vi "Test Data 2.vi"(8 "error in (no error)":errorcluster, 11 "Instrument.Lockin in":refnum<class "Instrument.Lockin.lvclass">) -> (0 "error out":errorcluster, 3 "Instrument.Lockin out":refnum<class "Instrument.Lockin.lvclass">)   [LabVIEW 2019]
uses:
  src/Instrument.Lockin/Instrument.Lockin.lvclass
  <vilib>/addons/_JKI Toolkits/Caraya/classes/Test/Test.lvclass
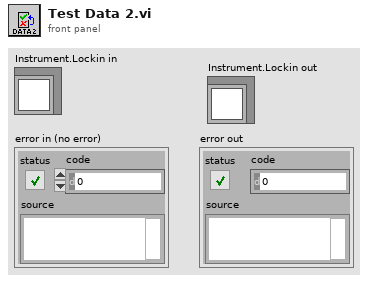
[diagram p1: front panel]
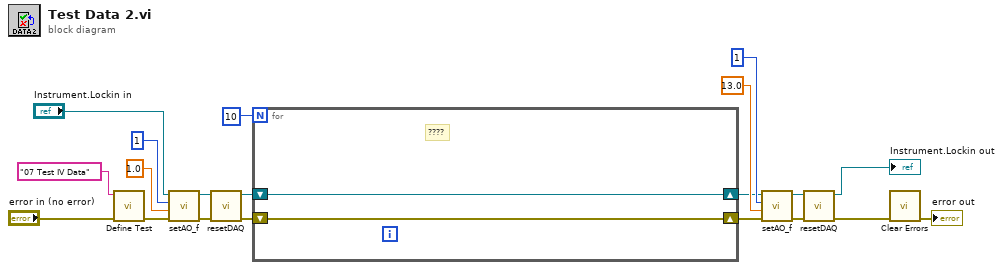
[diagram p0: block diagram]
diagram:
  n1 = call <vilib>:"Define Test.vi"("error in (no error)"="error in (no error)", "Label (VI Title)"="07 Test IV Data") -> ("error out"=w17:errorcluster)  [unwired: 8 in, 1 out]
  n2 = call-dynamic "setAO_f.vi"("error in (no error)"=w17, "Frequency (Hz)"=1.0, "AO Channel"=1, "Instrument.Lockin in"="Instrument.Lockin in") -> ("error out"=w9:errorcluster, "Instrument.Lockin out"=w8:refnum<class "Instrument.Lockin.lvclass">)  [unwired: 6 in]
  n3 = call-dynamic "resetDAQ.vi"("error in (no error)"=w9, "Instrument.Lockin in"=w8) -> ("error out"=w7:errorcluster, "Instrument.Lockin out"=w6:refnum<class "Instrument.Lockin.lvclass">)  [unwired: 8 in]
  n4 = for {
    N: 10 -> [_]
    shift-right: [w21] -> w11
    shift-left: w7 -> [w21]
    shift-right: [w22] -> w10
    shift-left: w6 -> [w22]
    # "????"
  }
  n5 = call-dynamic "setAO_f.vi"("error in (no error)"=w11, "Frequency (Hz)"=13.0, "AO Channel"=1, "Instrument.Lockin in"=w10) -> ("error out"=w4:errorcluster, "Instrument.Lockin out"=w3:refnum<class "Instrument.Lockin.lvclass">)  [unwired: 6 in]
  n6 = call-dynamic "resetDAQ.vi"("error in (no error)"=w4, "Instrument.Lockin in"=w3) -> ("error out"=w1:errorcluster, "Instrument.Lockin out"=→"Instrument.Lockin out":refnum<class "Instrument.Lockin.lvclass">)  [unwired: 8 in]
  n7 = call <vilib>:"Clear Errors.vi"("error in (no error)"=w1) -> ("error out"=→"error out":errorcluster)  [unwired: 5 in, 1 out]
